vi "Test Synchronize DAQ.vi"() -> ()   [LabVIEW 2019, in "DAQmx.lvclass"]
uses:
  DAQmx.lvclass
  DAQmx.lvclass/DAQmx.ctl
  <vilib>/measure/NI_MABase.lvlib
  <vilib>/DAQmx/write.llb/DAQmx Write (Analog 1D Wfm NChan NSamp).vi
  <vilib>/DAQmx/read.llb/DAQmx Read (Analog 1D Wfm NChan NSamp).vi
  typedefs/DAQ.Config.AI.Coupling--enum.ctl
  typedefs/DAQ.Config.AI.Range--enum.ctl
  typedefs/DAQ.Config.Device Type--enum.ctl
  typedefs/DAQ.Config.AI--Cluster.ctl
  typedefs/DAQ.Config.AO.Range--enum.ctl
  typedefs/DAQ.Config.AO--Cluster.ctl
  typedefs/DAQ.Config.Timing.Sampling--Cluster.ctl
panel:
  out "Waveform Graph":waveform(dbl)[](graph)
  in  "stop":bool
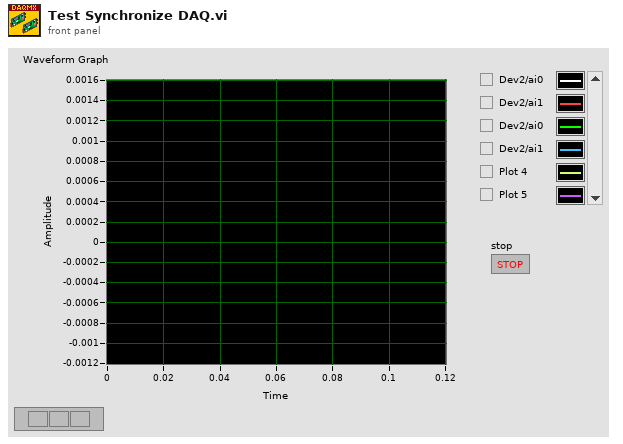
[diagram p1: front panel]
types:
  T1 = typedef "DAQmx.lvclass/DAQ.Config.Timing.Sampling--Cluster.ctl" = cluster{"Fs":dbl, "#s":i32}
  T2 = typedef "DAQmx.lvclass/DAQ.Config.AO--Cluster.ctl" = cluster{"Channels":tag, "Range":T3, "output terminal configuration":i32, "Type":T4}
  T3 = typedef "DAQmx.lvclass/DAQ.Config.AO.Range--enum.ctl" = enum16{"±0.1", "±1.0", "±10.0", ""}
  T4 = typedef "DAQmx.lvclass/DAQ.Config.Device Type--enum.ctl" = enum16{"None", "USB-4431", "PXI-446x"}
  T5 = typedef "DAQmx.lvclass/DAQ.Config.AI--Cluster.ctl" = cluster{"Channels":tag, "Coupling":T6, "Range":T7, "input terminal configuration":i32, "Type":T4}
  T6 = typedef "DAQmx.lvclass/DAQ.Config.AI.Coupling--enum.ctl" = u16
  T7 = typedef "DAQmx.lvclass/DAQ.Config.AI.Range--enum.ctl" = enum16{"±0.316", "±1.00", "±3.16", "±10.0", "±31.6", "±42.4", ""}
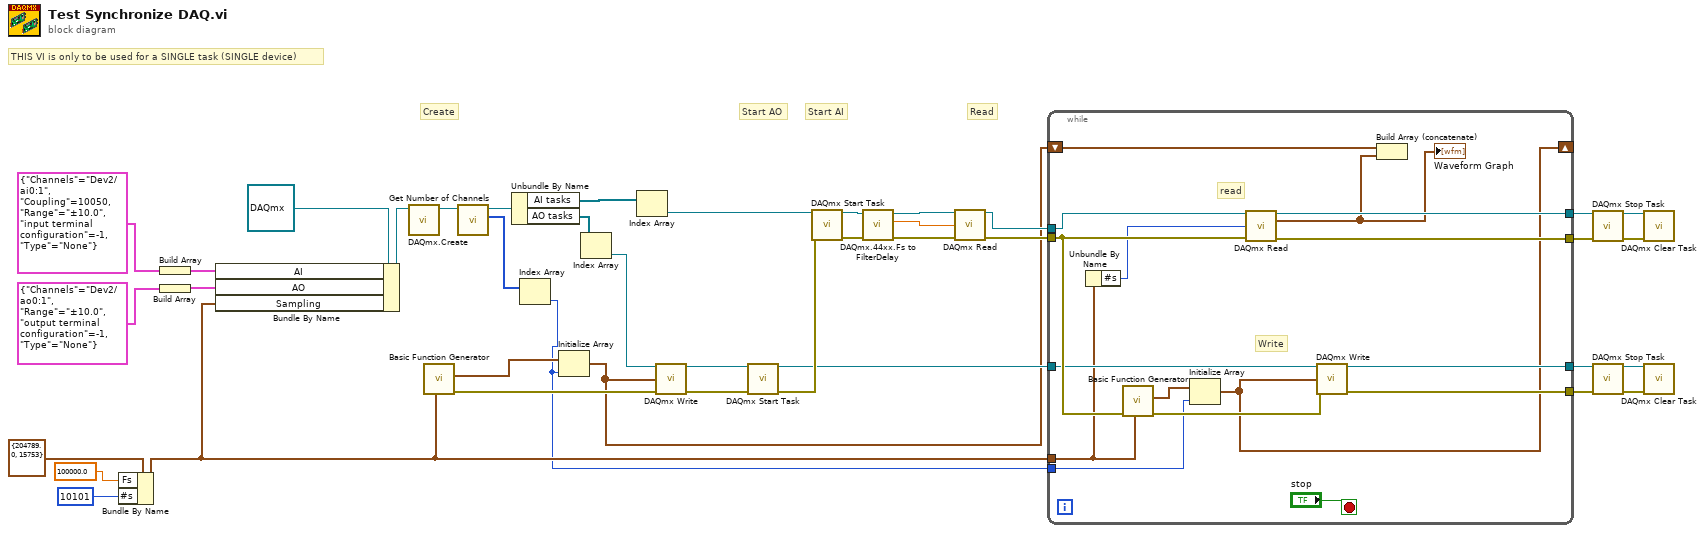
[diagram p0: block diagram]
diagram:
  # "THIS VI is only to be used for a SINGLE task (SINGLE device)"
  # "Read"
  # "Start AI"
  # "Start AO"
  # "Create"
  n1 = Bundle By Name(cluster=T1 {"Fs"=204789.0, "#s"=15753} ("Configuration.Sampling.Sampling"), "Fs"=100000.0, "#s"=10101) -> (w11:T1)
  n2 = Build Array(T5 {"Channels"="Dev2/ai0:1", "Coupling"=10050, "Range"=enum."±10.0", "input terminal configuration"=-1, "Type"=enum."None"} ("AI.Config")) -> (w6:T5[])
  n3 = Build Array(T2 {"Channels"="Dev2/ao0:1", "Range"=enum."±10.0", "output terminal configuration"=-1, "Type"=enum."None"} ("AO.config")) -> (w5:T2[])
  n4 = Bundle By Name(cluster=refnum<class "DAQmx.lvclass"> refnum ("DAQmx in"), "AI"=w6, "AO"=w5, "Sampling"=w11) -> (w15:refnum<class "DAQmx.lvclass">)
  n5 = call "DAQmx.Create.vi"("DAQmx in"=w15) -> ("DAQmx out"=w10:refnum<class "DAQmx.lvclass">)  [unwired: 9 in, 1 out]
  n6 = call <vilib>:"Basic Function Generator.vi"("sampling info"=w11) -> ("error out"=w36:errorcluster, "signal out"=w8:waveform(dbl))  [unwired: 8 in, 1 out]
  n7 = call "Get Number of Channels.vi"("DAQmx in"=w10) -> ("Channels each Device"=w7:u32[], "DAQmx out"=w9:refnum<class "DAQmx.lvclass">)  [unwired: 7 in, 2 out]
  n8 = Unbundle By Name(w9) -> ("AI tasks"=w34:refnum<k21>[], "AO tasks"=w40:refnum<k21>[])
  n9 = Index Array(array=w7) -> (element=w1:u32)  [unwired: 1 in]
  n10 = Initialize Array(w8, w1) -> (w4:waveform(dbl)[])
  n11 = Index Array(array=w40) -> (element=w39:refnum<k21>)  [unwired: 1 in]
  n12 = Index Array(array=w34) -> (element=w35:refnum<k21>)  [unwired: 1 in]
  n13 = call-poly <vilib>:"DAQmx Write.vi"("task/channels in"=w39, "data"=w4, "error in"=w36) -> ("task out"=w38:refnum<k21>, "error out"=w37:errorcluster)  [unwired: 10 in, 1 out]
  n14 = call <vilib>:"DAQmx Start Task.vi"("task/channels in"=w38, "error in"=w37) -> ("task out"=w14:refnum<k21>, "error out"=w29:errorcluster)  [unwired: 12 in]
  n15 = call <vilib>:"DAQmx Start Task.vi"("task/channels in"=w35, "error in"=w29) -> ("task out"=w32:refnum<k21>, "error out"=w33:errorcluster)  [unwired: 12 in]
  n16 = call "DAQmx.44xx.Fs to FilterDelay.vi"("error in (no error)"=w33, "Refnum in"=w32) -> ("error out"=w12:errorcluster, "ADC Delay (samples)"=w31:dbl, "Refnum out"=w30:refnum<k21>)  [unwired: 5 in, 2 out]
  n17 = call-poly <vilib>:"DAQmx Read.vi"("task/channels in"=w30, "number of samples per channel"=w31, "error in"=w12) -> ("task out"=w28:refnum<k21>, "error out"=w27:errorcluster)  [unwired: 10 in, 1 out]
  n18 = while {
    tunnel: w28 -> [w56]
    tunnel: w27 -> [w55]
    tunnel: w14 -> [w53]
    tunnel: w11 -> [w46]
    tunnel: [w52] -> w26
    tunnel: [w51] -> w25
    tunnel: [w50] -> w20
    tunnel: [w47] -> w19
    shift-right: [w43] -> _
    shift-left: w4 -> [w45]
    tunnel: w1 -> [w44]
    stop <- "stop" stop-if-true
    # "read"
    # "Write"
    n19 = Unbundle By Name(w46) -> ("#s"=w49:i32)
    n20 = call <vilib>:"Basic Function Generator.vi"("sampling info"=w46, "error in (no error)"=w55) -> ("error out"=w48:errorcluster, "signal out"=w41:waveform(dbl))  [unwired: 7 in, 1 out]
    n21 = Initialize Array(w41, w44) -> (w43:waveform(dbl)[])
    n22 = call-poly <vilib>:"DAQmx Read.vi"("task/channels in"=w56, "number of samples per channel"=w49, "error in"=w55) -> ("task out"=w52:refnum<k21>, "data"=w42:waveform(dbl)[], "error out"=w51:errorcluster)  [unwired: 10 in]
    "Waveform Graph" <- w42
    n23 = call-poly <vilib>:"DAQmx Write.vi"("task/channels in"=w53, "data"=w43, "error in"=w48) -> ("task out"=w50:refnum<k21>, "error out"=w47:errorcluster)  [unwired: 10 in, 1 out]
    n24 = Build Array (concatenate)(w45, w42) -> ()  [unwired: 1 out]
  }
  n25 = call <vilib>:"DAQmx Stop Task.vi"("task/channels in"=w26, "error in"=w25) -> ("task out"=w23:refnum<k21>, "error out"=w24:errorcluster)  [unwired: 12 in]
  n26 = call <vilib>:"DAQmx Stop Task.vi"("task/channels in"=w20, "error in"=w19) -> ("task out"=w22:refnum<k21>, "error out"=w21:errorcluster)  [unwired: 12 in]
  n27 = call <vilib>:"DAQmx Clear Task.vi"("task in"=w23, "error in"=w24) -> ()  [unwired: 13 in, 1 out]
  n28 = call <vilib>:"DAQmx Clear Task.vi"("task in"=w22, "error in"=w21) -> ()  [unwired: 13 in, 1 out]
